vi "NXTServo-Dual.vi"() -> ()   [LabVIEW 2009]
uses:
  <vilib>/NXT/Block Support/NXT_InputPort.ctl
  <vilib>/NXT/Subs/LVHSConnector.ctl
  mindsensors.com LVEE Toolkit/Dual/NXTServo-DM.vi
panel:
  out "Output of NXTServo":cluster{"Voltage":u8, "Status":bool}
  in  "Input of NXTServo":T1={"Servo Number"=1, "Position"=1500, "Speed"=0} {"Speed" step=1 scale=0.0..255.0; "Position" min=500 max=2500 step=1 scale=500.0..2500.0; "Servo Number" min=1 max=8 step=1}
  in  "NXT":T2={"error"={"status"=FALSE, "code"=0, "source"=""}, "address"="", "NXT #"=0, "Show Error"=FALSE, "Connection"=4} {"Connection" items=["USB", "Bluetooth", "USB then Bluetooth", "Last Connection", "Preference"]}
  out "NXT dup":T2={"error"={"status"=FALSE, "code"=0, "source"=""}, "address"="", "NXT #"=0, "Show Error"=FALSE, "Connection"=4} caption="NXT" {"Connection" items=["USB", "Bluetooth", "USB then Bluetooth", "Last Connection", "Preference"]}
  in  "Input Port":T3 items=["Port 1", "Port 2", "Port 3", "Port 4"]
  in  "stop":bool
  # "mindsensors.com\nCopyright (c) 2009 by mindsensors.com\nEmail: info (<at>) mindsensors (<dot>) com\n\nThis program is free software. You can redistribute it and/or modify\nit under the terms of the GNU General Public License as published by\nthe Free Software Foundation; version 3 of the License.\nRead the license at: http://www.gnu.org/licenses/gpl.txt"
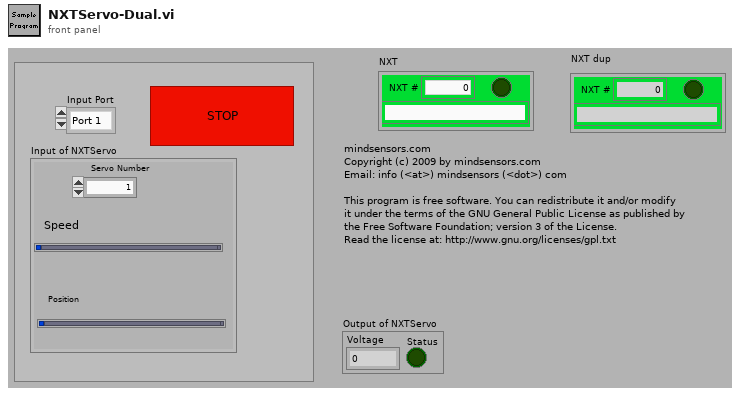
[diagram p1: front panel]
types:
  T1 = cluster{"Servo Number":u8, "Position":u16, "Speed":u8}
  T2 = typedef "LVHSConnector.ctl" = cluster{"error":errorcluster, "address":string, "NXT #":i32, "Show Error":bool, "Connection":u16}
  T3 = typedef "NXT_InputPort.ctl" = u8
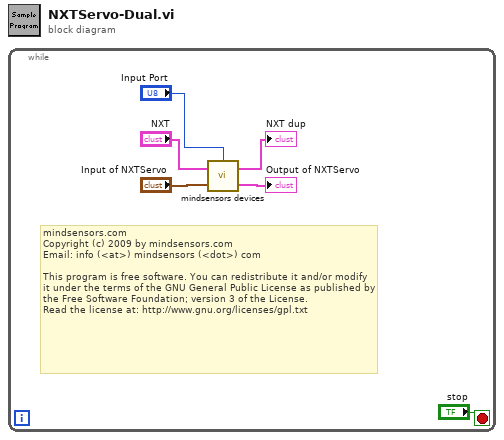
[diagram p0: block diagram]
diagram:
  n1 = while {
    stop <- "stop" stop-if-true
    # "mindsensors.com\nCopyright (c) 2009 by mindsensors.com\nEmail: info (<at>) mindsensors (<dot>) com\n\nThis program is free software. You can redistribute it and/or modify\nit under the terms of the GNU General Public License as published by\nthe Free Software Foundation; version 3 of the License.\nRead the license at: http://www.gnu.org/licenses/gpl.txt"
    n2 = call-poly "mindsensors devices.vi"("Input of NXTServo"="Input of NXTServo", "NXT"="NXT", "Input Port"="Input Port") -> ("Output of NXTServo"=→"Output of NXTServo":cluster{"Voltage":u8, "Status":bool}, "NXT dup"=→"NXT dup":T2)
  }
